vi "Reduce_Plot_Size.vi"(9 "Array":cluster{dbl[], dbl[]}[](array[cluster]), 10 "Width":i32, 11 "X Scale.Range":T1) -> (3 "Array 2":cluster{dbl[], dbl[]}[](array[cluster]))   [LabVIEW 2016]
uses:
  <vilib>/Utility/miscctls.llb/LVRangeTypeDef.ctl
panel:
  out "Numeric":dbl format="%#_13g"
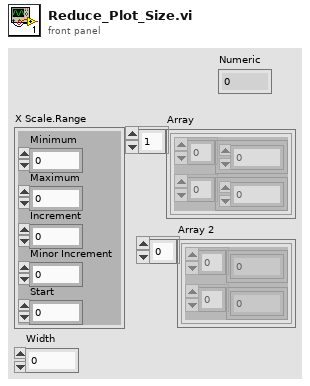
[diagram p1: front panel]
types:
  T1 = typedef "LVRangeTypeDef.ctl" = cluster{"Minimum":dbl, "Maximum":dbl, "Increment":dbl, "Minor Increment":dbl, "Start":dbl}
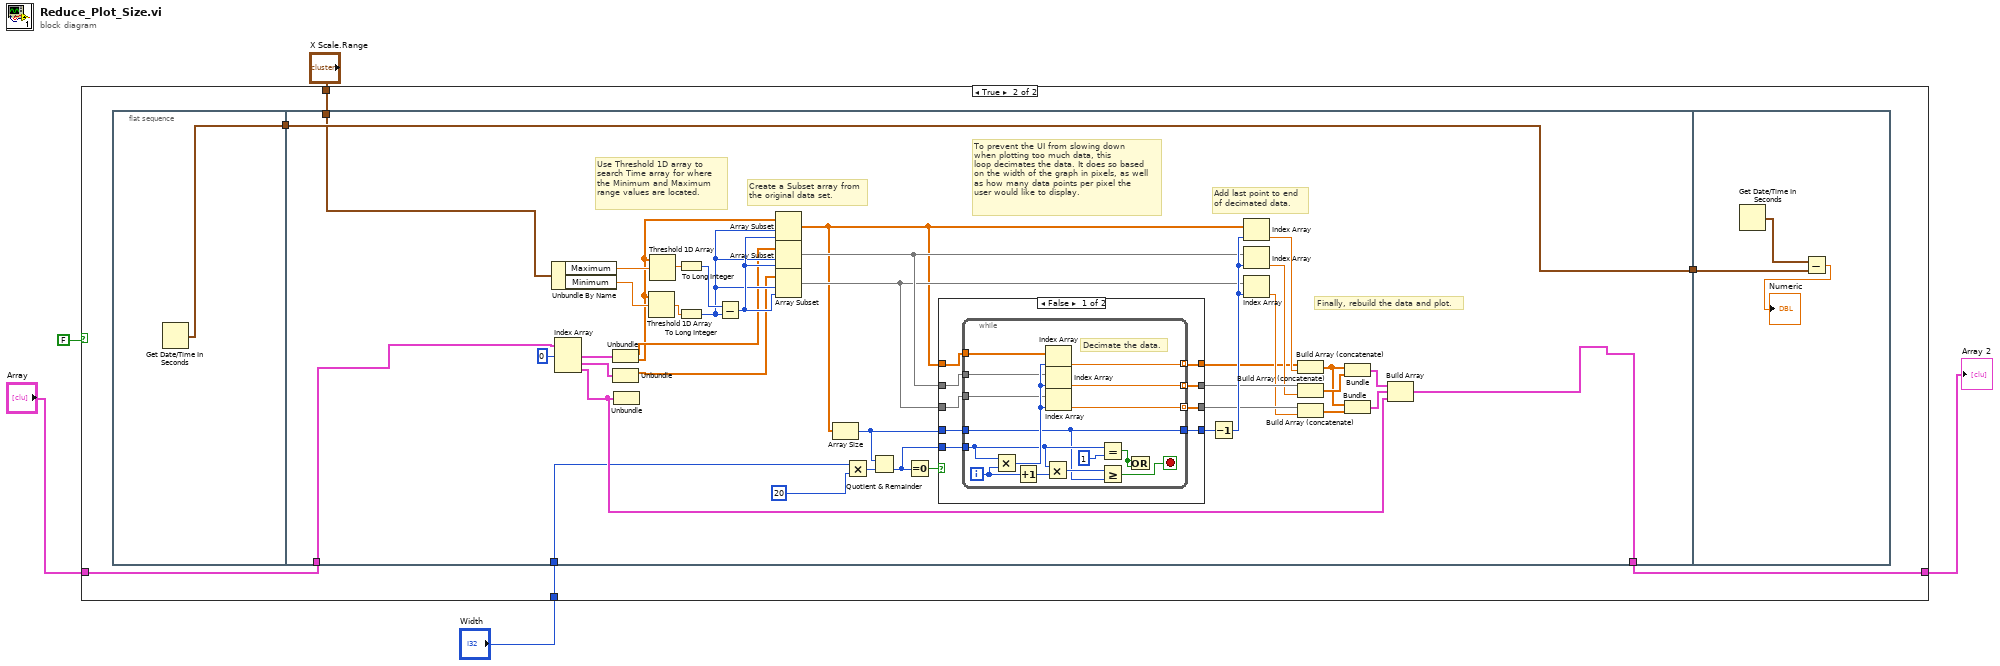
[diagram p0: block diagram]
diagram:
  n1 = case shown="True" FALSE {
    tunnel: [w6 w10] -> w5
    tunnel: "Array" -> [w6 w9]
    tunnel: "X Scale.Range" -> [_ w8]
    tunnel: "Width" -> [_ w7]
    frame False {
    }
    frame True {
      n2 = flat-sequence {
        tunnel: [w13] -> w12
        tunnel: [w21] -> w11
        tunnel: w12 -> [w21]
        tunnel: [w20] -> w10
        tunnel: w9 -> [w19]
        tunnel: w8 -> [w18]
        tunnel: w7 -> [w17]
        tunnel: w11 -> [w83]
        frame #0 {
          n3 = Get Date/Time In Seconds() -> (seconds since 1Jan1904=w13:timestamp)
        }
        frame #1 {
          # "Add last point to end\nof decimated data."
          # "Finally, rebuild the data and plot."
          # "To prevent the UI from slowing down\nwhen plotting too much data, this\nloop decimates the data. It does so based\non the width of the graph in pixels, as well\nas how many data points per pixel the\nuser would like to display."
          # "Create a Subset array from\nthe original data set."
          # "Use Threshold 1D array to\nsearch Time array for where\nthe Minimum and Maximum\nrange values are located."
          n4 = Unbundle By Name(w18) -> ("Maximum"=w25:dbl, "Minimum"=w47:dbl)
          n5 = Index Array(array=w19, index #1=0 ("index")) -> (element #1=w52:cluster{dbl[], dbl[]}, element #2=w51:cluster{dbl[], dbl[]}, element #3=w22:cluster{dbl[], dbl[]})  [unwired: 2 in]
          n6 = Unbundle(w52) -> (w16:dbl[], w15:dbl[])
          n7 = Unbundle(w51) -> (w14:dbl[])  [unwired: 1 out]
          n8 = Unbundle(w22) -> ()  [unwired: 2 out]
          n9 = Threshold 1D Array(2:w47, 3:w15) -> (0:w45:dbl)  [unwired: 1 in]
          n10 = Threshold 1D Array(2:w25, 3:w15) -> (0:w46:dbl)  [unwired: 1 in]
          n11 = To Long Integer(number=w46) -> (32bit integer=w33:i32)
          n12 = To Long Integer(number=w45) -> (32bit integer=w32:i32)
          n13 = Subtract(x=w33, y=w32) -> (x-y=w48:i32)
          n14 = Array Subset(array=w15, index=w32, length=w48) -> (w26:dbl[])
          n15 = Array Subset(array=w16, index=w32, length=w48) -> (w42:dbl[])
          n16 = Array Subset(array=w14, index=w32, length=w48) -> (w27:dbl[])
          n17 = Array Size(array=w26) -> (size(s)=w31:i32)
          n18 = Multiply(x=w17, y=20) -> (x*y=w28:i32)
          n19 = Quotient & Remainder(x=w31, y=w28) -> (floor(x/y)=w24:i32)  [unwired: 1 out]
          n20 = Equal To 0?(x=w24) -> (x = 0?=w29:bool)
          n21 = case shown="False" w29 {
            tunnel: [w62 w78] -> w44
            tunnel: w26 -> [w61 w81]
            tunnel: w42 -> [w60 w80]
            tunnel: w27 -> [w59 w79]
            tunnel: [w58 w80] -> w41
            tunnel: [w57 w79] -> w40
            tunnel: w31 -> [w56 w78]
            tunnel: [w55 w81] -> w30
            tunnel: w24 -> [w54 _]
            frame False {
              n22 = while {
                tunnel: w61 -> [w74]
                tunnel: w60 -> [w68]
                tunnel: w59 -> [w72]
                tunnel: w56 -> [w65]
                tunnel: [w71] -> w55 mode=indexing
                tunnel: [w70] -> w58 mode=indexing
                tunnel: [w69] -> w57 mode=indexing
                tunnel: w54 -> [w67]
                tunnel: [w65] -> w62
                i -> [w77]
                stop <- w63 stop-if-true
                # "Decimate the data."
                n23 = Multiply(x=w67, y=w77) -> (x*y=w73:i32)
                n24 = Increment(x=w77) -> (x+1=w76:i32)
                n25 = Multiply(x=w67, y=w76) -> (x*y=w75:i32)
                n26 = Index Array(array=w74, index=w73) -> (element=w71:dbl)
                n27 = Index Array(array=w68, index=w73) -> (element=w70:dbl)
                n28 = Index Array(array=w72, index=w73) -> (element=w69:dbl)
                n29 = Equal?(x=w67, y=u32 1) -> (x = y?=w64:bool)
                n30 = Greater Or Equal?(x=w75, y=w65) -> (x >= y?=w63:bool)
                n31 = Or(x=w64, y=w64) -> ()  [unwired: 1 out]
              }
            }
            frame True {
            }
          }
          n32 = Decrement(x=w44) -> (x-1=w43:i32)
          n33 = Index Array(array=w26, index=w43) -> (element=w34:dbl)
          n34 = Index Array(array=w42, index=w43) -> (element=w39:dbl)
          n35 = Index Array(array=w27, index=w43) -> (element=w38:dbl)
          n36 = Build Array (concatenate)(w30, w34) -> (w35:dbl[])
          n37 = Build Array (concatenate)(w41, w39) -> (w37:dbl[])
          n38 = Build Array (concatenate)(w40, w38) -> (w36:dbl[])
          n39 = Bundle(w35, w37) -> (w50:cluster{dbl[], dbl[]})  [unwired: 1 in]
          n40 = Bundle(w35, w36) -> (w49:cluster{dbl[], dbl[]})  [unwired: 1 in]
          n41 = Build Array(w50, w49, w22) -> (w20:cluster{dbl[], dbl[]}[])
        }
        frame #2 {
          n42 = Get Date/Time In Seconds() -> (seconds since 1Jan1904=w84:timestamp)
          n43 = Subtract(x=w84, y=w83) -> (x-y=→"Numeric":dbl)
        }
      }
    }
  }
  "Array 2" <- w5
